vi "Test_TimeoutStop_SubstituteLastMessage_LastMessageExecutedOnce.vi"(8 "error in (no error)":errorcluster, 11 "TestCase in":refnum<class "TestMessageCycle.lvclass">) -> (0 "error out":errorcluster, 3 "TestCase out":refnum<class "TestMessageCycle.lvclass">)   [LabVIEW 2017, in "TestMessageCycle.lvclass"]
uses:
  TestMessageCycle.lvclass
  <vilib>/ActorFramework/Message/Message.lvclass
  Source/MessageCycle/Message Cycle Notifications.ctl
  Source/MessageCycle/MessageCycle.lvclass/MessageCycle.ctl
  <vilib>/ActorFramework/Message Enqueuer/Message Enqueuer.lvclass/Message Enqueuer.ctl
  1b07eade-a78c-42fd-a35c-617bb70b86e5.vi
  <vilib>/ActorFramework/Message Enqueuer/Enqueue.vi
  Doubles/MessageCountsExecutions/MessageCountsExecutions.lvclass
  C:/Program Files (x86)/National Instruments/LabVIEW 2017/vi.lib/ActorFramework/Message/Message.lvclass
  Doubles/ActorCountsMessageCycles/ActorCountsMessageCycles.lvclass
  C:/Program Files (x86)/National Instruments/LabVIEW 2017/vi.lib/ActorFramework/Actor/Actor.lvclass
  Source/MessageCycle/MessageCycle.lvclass
  <vilib>/ActorFramework/Stop Msg/Stop Msg.lvclass
  Source/MessageCycle/Launch Deferred Timeout Notifier.vi
  <vilib>/ActorFramework/Message Priority Queue/Priority Enqueue.vi
  <vilib>/ActorFramework/Actor/Actor.lvclass
panel:
  out "\"Last Message\" Executions":u32
  out "Cyclic Messages Received":u32
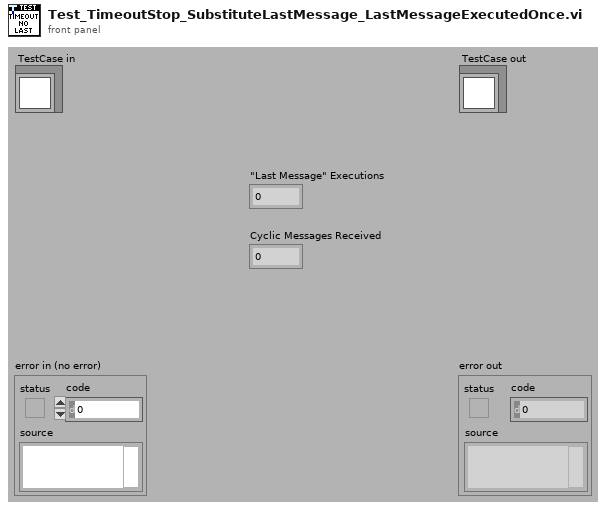
[diagram p1: front panel]
types:
  T1 = typedef "MessageCycle.lvclass/Message Cycle Notifications.ctl" = enum16{"Process Final Copy and Stop", "Stop Immediately", "Substitute Last Message and Stop"}
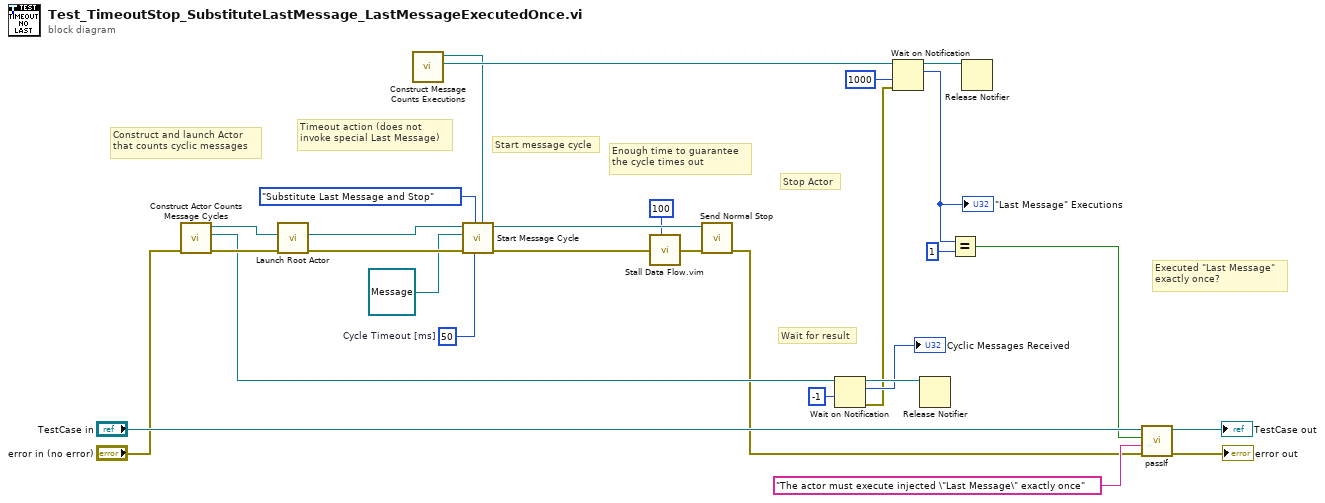
[diagram p0: block diagram]
diagram:
  w5 = 50  # Cycle Timeout [ms]
  # "Enough time to guarantee\nthe cycle times out"
  # "Timeout action (does not\ninvoke special Last Message)"
  # "Wait for result"
  # "Stop Actor"
  # "Start message cycle"
  # "Executed \"Last Message\"\nexactly once?"
  # "Construct and launch Actor\nthat counts cyclic messages"
  n1 = call "Construct Actor Counts Message Cycles.vi"("error in (no error)"="error in (no error)") -> ("error out"=w19:errorcluster, "Final Count"=w18:refnum<notifier>, "ActorCountsMessageCycles"=w21:refnum<class "ActorCountsMessageCycles.lvclass">)  [unwired: 8 in]
  n2 = call <vilib>:"Launch Root Actor.vi"("error in (no error)"=w19, "Actor"=w21) -> ("error out"=w29:errorcluster, "Actor's Enqueuer"=w25:refnum<class "Message Enqueuer.lvclass">)  [unwired: 8 in]
  n3 = call "Construct Message Counts Executions.vi"() -> ("Message Executions"=w8:refnum<notifier>, "CyclicMessageCountsCycles out"=w3:refnum<class "MessageCountsExecutions.lvclass">)  [unwired: 9 in, 1 out]
  n4 = call "Start Message Cycle.vi"("Last Message"=w3, "Cycle Timeout [ms] (-1)"=w5, "Timeout Action"=Message_Cycle_Notifications."Substitute Last Message and Stop", "error in (no error)"=w29, "Message"=refnum<class "Message.lvclass"> refnum, "Message Enqueuer"=w25) -> ("error out"=w13:errorcluster, "Message Enqueuer out"=w24:refnum<class "Message Enqueuer.lvclass">)  [unwired: 3 in, 1 out]
  n5 = call "Stall Data Flow.vim"("value in"=w13, "milliseconds to wait"=u32 100) -> ("value out"=w12:errorcluster)  [unwired: 1 out]
  n6 = call <vilib>:"Send Normal Stop.vi"("error in (no error)"=w12, "Message Enqueuer"=w24) -> ("error out"=w15:errorcluster)  [unwired: 9 in]
  n7 = Wait on Notification(notifier=w18, timeout in ms (-1)=-1) -> (notifier out=w16:refnum<notifier>, notification=→"Cyclic Messages Received":u32, error out=w9:errorcluster)  [unwired: 2 in, 1 out]
  n8 = Wait on Notification(notifier=w8, timeout in ms (-1)=1000, error in (no error)=w9) -> (notifier out=w7:refnum<notifier>, notification=w2:u32)  [unwired: 1 in, 2 out]
  "\"Last Message\" Executions" <- w2
  n9 = Release Notifier(notifier=w16) -> ()  [unwired: 2 in, 3 out]
  n10 = Equal?(x=w2, y=u32 1) -> (x = y?=w23:bool)
  n11 = Release Notifier(notifier=w7) -> ()  [unwired: 2 in, 3 out]
  n12 = call-dynamic "passIf.vi"("error in (no error)"=w15, "message (\"\")"="The actor must execute injected \"Last Message\" exactly once" ("message (\"\")"), "pass"=w23, "TestCase in"="TestCase in") -> ("error out"=→"error out":errorcluster, "TestCase out"=→"TestCase out":refnum<class "TestMessageCycle.lvclass">)  [unwired: 6 in]
